vi "SVT Power Spectrum Subset.vi"   [LabVIEW 2017]
doc: "Computes a subset of the power spectrum of <B>scaled signal [EU]</B>. The subset is defined by <B>frequency range</B>. Each block of data corresponds to a single FFT block and has to be passed individually to this VI. You can use this polymorphic VI to analyze signals from a single channel or from N channels. The data type you wire to the <B>scaled signal [EU]</B> input determines the polymorphic instance to use."
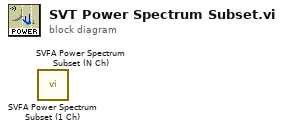
[diagram p0: block diagram]
diagram:
  n1 = call <vilib>:"SVFA Power Spectrum Subset (1 Ch).vi"() -> ()  [unwired: 14 in, 6 out]
  n2 = call <vilib>:"SVFA Power Spectrum Subset (N Ch).vi"() -> ()  [unwired: 14 in, 6 out]
